vi "DoubleAsValue.vi"(8 "error in":errorcluster, 11 "scalar value (double)":dbl) -> (0 "error out":errorcluster, 3 "scalar string":string)   [LabVIEW 2014]
doc: "Fromat a LV double as an XML-RPC double"
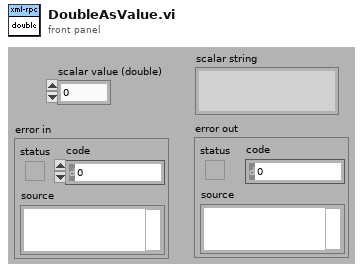
[diagram p1: front panel]
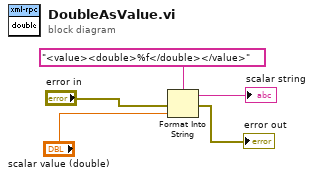
[diagram p0: block diagram]
diagram:
  n1 = Format Into String(format string="<value><double>%f</double></value>", error in="error in", "scalar value (double)") -> (resulting string=→"scalar string":string, error out=→"error out":errorcluster)  [unwired: 1 in]
